vi "IndexArray.vi"(9 "index":i32, 11 "read buffer":string) -> (1 "Numeric":u8, 3 "String":string)   [LabVIEW 2011]
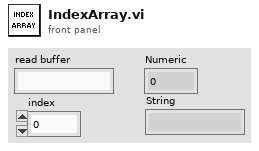
[diagram p1: front panel]
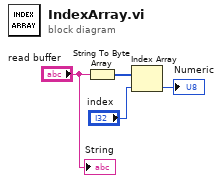
[diagram p0: block diagram]
diagram:
  n1 = String To Byte Array(string="read buffer") -> (unsigned byte array=w2:u8[])
  n2 = Index Array(array=w2, index="index") -> (element=→"Numeric":u8)
  "String" <- "read buffer"
